vi "Build Insert Query.vi"(7 "Schema Name":string, 8 "error in (no error)":errorcluster, 9 "Data":string[][](array[string]), 10 "Column Names":string[](array[string]), 11 "Table Name":string) -> (0 "error out":errorcluster, 3 "SQL":string caption="SQL+ (Col[]) VALUES (?[])")   [LabVIEW 2023, in "HardwareAbstractionLayer_LVOOP.lvlib" / "Database.lvclass"]
uses:
  Database.lvclass
  <vilib>/Utility/error.llb/Trim Whitespace One-Sided.vi
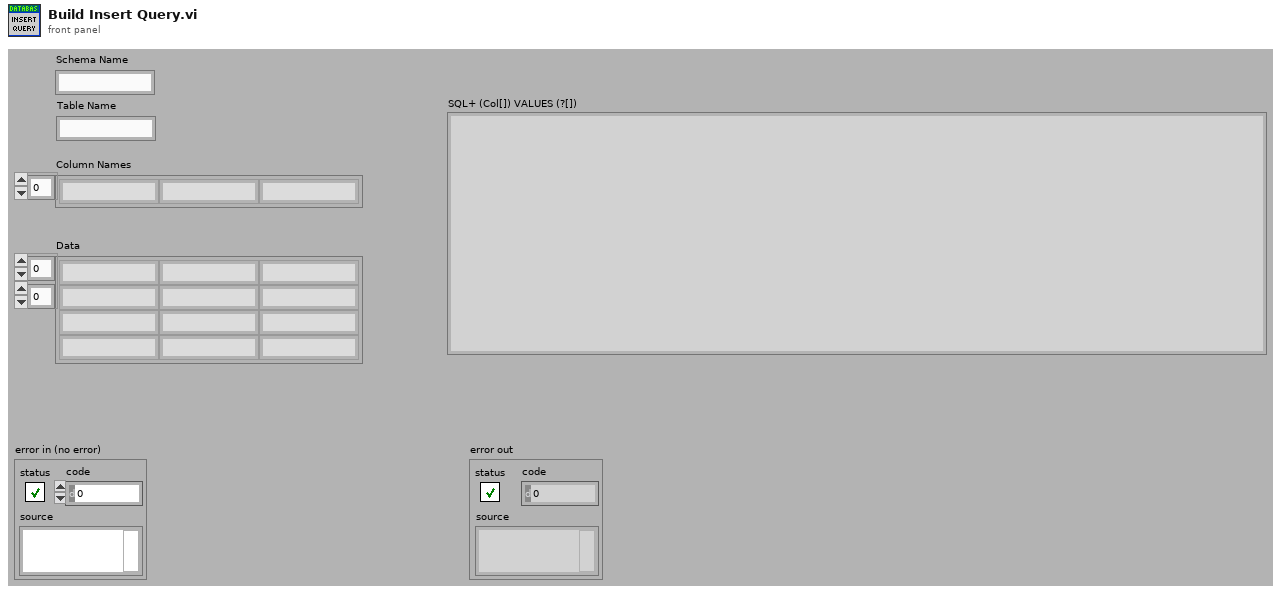
[diagram p1: front panel]
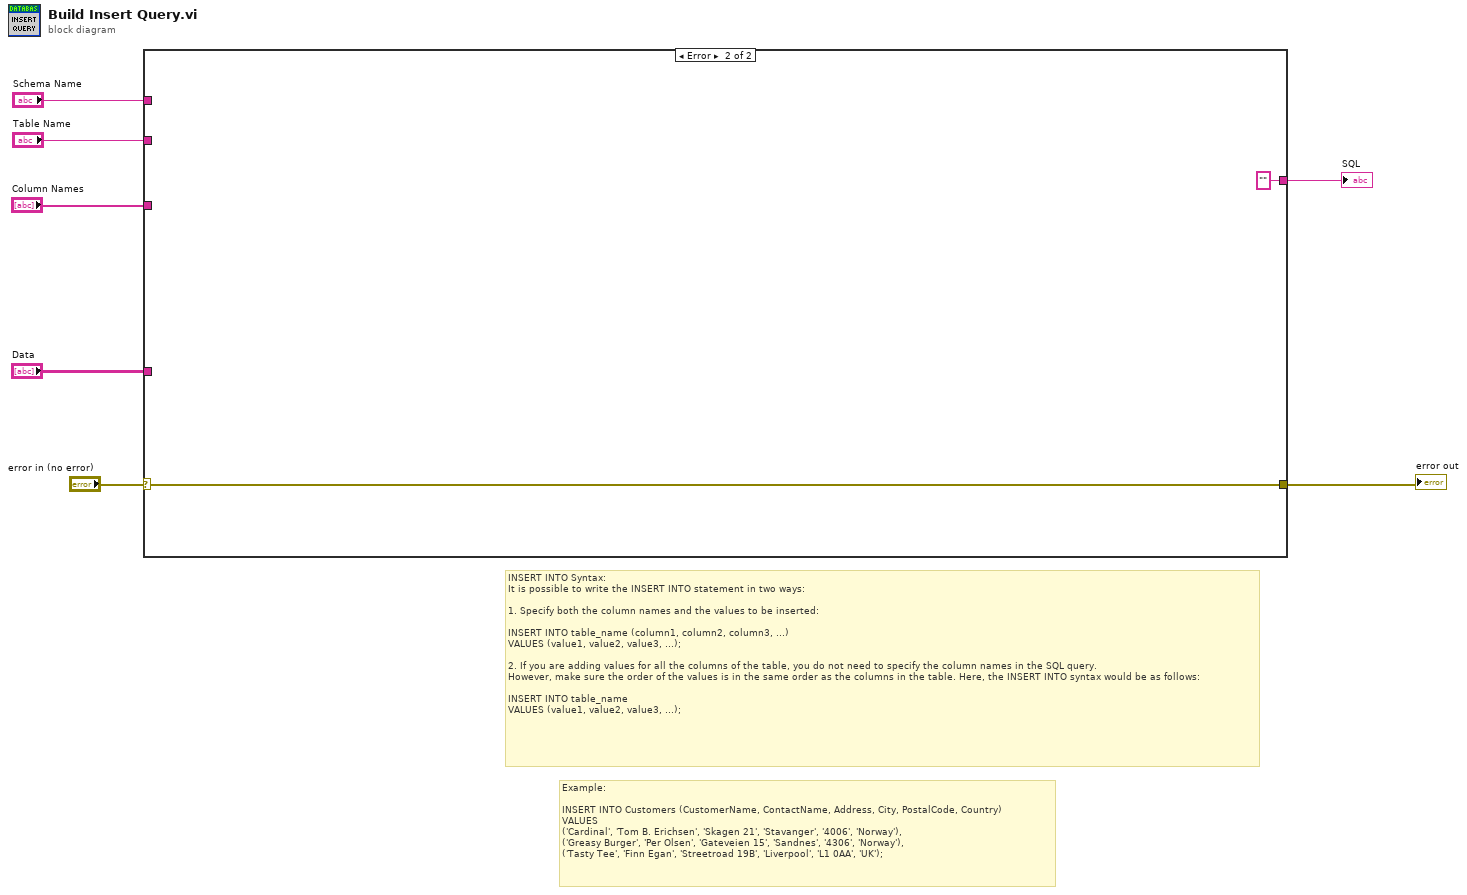
[diagram p0: block diagram]
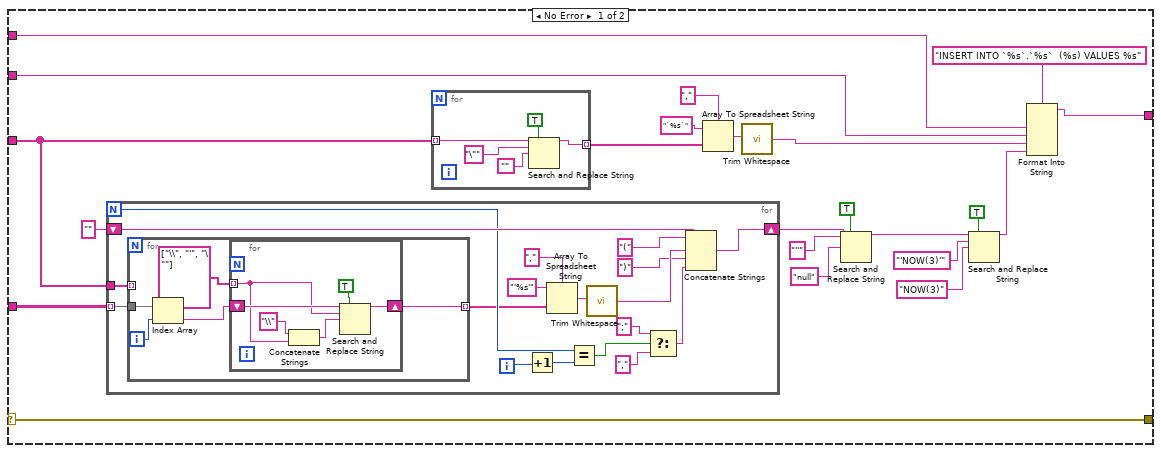
[diagram p2: hidden frame]
diagram:
  # "Example:\n\nINSERT INTO Customers (CustomerName, ContactName, Address, City, PostalCode, Country)\nVALUES\n('Cardinal', 'Tom B. Erichsen', 'Skagen 21', 'Stavanger', '4006', 'Norway'),\n('Greasy Burger', 'Per Olsen', 'Gateveien 15', 'Sandnes', '4306', 'Norway'),\n('Tasty Tee', 'Finn Egan', 'Streetroad 19B', 'Liverpool', 'L1 0AA', 'UK');"
  # "INSERT INTO Syntax: \nIt is possible to write the INSERT INTO statement in two ways:\n\n1. Specify both the column names and the values to be inserted:\n\nINSERT INTO table_name (column1, column2, column3, ...)\nVALUES (value1, value2, value3, ...);\n\n2. If you are adding values for all the columns of the table, you do not need to specify the column names in the SQL query. \nHowever, make sure the order of the values is in the same order as the columns in the table. Here, the INSERT INTO syntax would be as follows:\n\nINSERT INTO table_name\nVALUES (value1, value2, value3, ...);"
  n1 = case shown="Error" "error in (no error)" {
    selector: "error in (no error)" -> [w29 w65]
    tunnel: [w29 w65] -> w6
    tunnel: "Column Names" -> [w9 _]
    tunnel: "Data" -> [w24 _]
    tunnel: "Table Name" -> [w21 _]
    tunnel: "Schema Name" -> [w15 _]
    tunnel: [w8 ""] -> w1
    frame No Error {
      n2 = for {
        N -> [w45]
        tunnel: w24 -> [w37] mode=indexing
        shift-right: [w49] -> w19
        shift-left: "" -> [w46]
        tunnel: w9 -> [w35]
        i -> [w44]
        n3 = for {
          tunnel: w37 -> [w57]
          tunnel: [w53] -> w36 mode=indexing
          tunnel: w35 -> [_] mode=indexing
          i -> [w56]
          n4 = Index Array(array=w57, index=w56) -> (element=w55:string)
          n5 = for {
            tunnel: string[] ["\\", "'", "\""] -> [w58] mode=indexing
            shift-right: [w61] -> w53
            shift-left: w55 -> [w62]
            n6 = Concatenate Strings("\\", w58) -> (w59:string)
            n7 = Search and Replace String(replace all?=TRUE ("replace all? (F)"), input string=w62, search string=w58, replace string=w59) -> (result string=w61:string)  [unwired: 4 in, 3 out]
          }
        }
        n8 = Increment(x=w44) -> (x+1=w43:i32)
        n9 = Array To Spreadsheet String(delimiter (Tab)=",", array=w36, 3:"'%s'" ("format string")) -> (spreadsheet string=w52:string)
        n10 = Equal?(x=w45, y=w43) -> (x = y?=w42:bool)
        n11 = call <vilib>:"Trim Whitespace.vi"("string"=w52) -> ("trimmed string"=w50:string)  [unwired: 1 in]
        n12 = Select(t=";" ("string"), s=w42, f="," ("string")) -> (s? t:f=w40:string)
        n13 = Concatenate Strings(w46, "(" ("string"), w50, ")" ("string"), w40) -> (w49:string)
      }
      n14 = for {
        tunnel: w9 -> [w34] mode=indexing
        tunnel: [w33] -> w20 mode=indexing
        n15 = Search and Replace String(replace all?=TRUE ("replace all? (F)"), input string=w34, search string="\"", replace string="") -> (result string=w33:string)  [unwired: 4 in, 3 out]
      }
      n16 = Array To Spreadsheet String(delimiter (Tab)=",", array=w20, 3:"`%s`" ("format string")) -> (spreadsheet string=w26:string)
      n17 = call <vilib>:"Trim Whitespace.vi"("string"=w26) -> ("trimmed string"=w22:string)  [unwired: 1 in]
      n18 = Search and Replace String(replace all?=TRUE ("replace all? (F)"), input string=w19, search string="''", replace string="null") -> (result string=w11:string)  [unwired: 4 in, 3 out]
      n19 = Search and Replace String(replace all?=TRUE ("replace all? (F)"), input string=w11, search string="'NOW(3)'", replace string="NOW(3)") -> (result string=w10:string)  [unwired: 4 in, 3 out]
      n20 = Format Into String(format string="INSERT INTO `%s`.`%s`  (%s) VALUES %s", w15, w21, w22, w10) -> (resulting string=w8:string)  [unwired: 2 in, 1 out]
    }
    frame Error {
    }
  }
  "error out" <- w6
  "SQL" <- w1
